vi "FDR.vi"(0 "System no.":i32=1 min=1 step=1, 1 "Board":i32=1 min=1 max=5 step=1, 2 "Routinename":string, 3 "Scan axis settings":T7={"Scan axis"="", "Range scan axis"=0.1, "Set Mid. pos?"=FALSE, "Mid. pos. scan axis"=0.1} {"Mid. pos. scan axis" format="%.4f"; "Range scan axis" format="%.4f"}, 4 "Step axis settings":T6={"Step axis"="", "Range step axis"=0.1, "Set Mid. pos?"=FALSE, "Mid. pos. step axis"=0.1} {"Mid. pos. step axis" format="%.4f"; "Range step axis" format="%.4f"}, 5 "error in":errorcluster, 6 "Threshold level":dbl=1.0 format="%.3f", 7 "Frequency settings":cluster{"Set frequency?":bool, "Frequency":dbl}={"Set frequency?"=FALSE, "Frequency"=10.0} {"Frequency" format="%.3f"}, 8 "Velocity settings":cluster{"Set velocity?":bool, "Velocity":dbl}={"Set velocity?"=FALSE, "Velocity"=0.1} {"Velocity" format="%.4f"}, 9 "Stop position option settings":T5, 10 "Target type settings":T4, 11 "Min. relative input level (MIIL) settings":T2={"Set min. input level?"=FALSE, "MIIL"=10.0}, 12 "Centroid method settings":T3, 13 "Max. relative input level (MAIL) settings":T1={"Set max. input level?"=FALSE, "MAIL"=80.0}) -> (19 "error out":errorcluster)   [LabVIEW 2026]
doc: "Defines a fast alignment area scan routine. Use FRS to start the routine and FRR? to read out the results of the routine. \n\nC-887, E-712, E-727.AS:"
panel:
  # "Defines a fast alignment raster scan routine. Use FRS to start the routine\nand FRR? to read out the results of the routine."
  # "If Yes:"
  # "If Yes:"
  # "If Yes:"
  # "If Yes:"
  # "If Yes:"
  # "If Yes:"
  # "If Yes:"
  # "If Yes:"
  # "If Yes:"
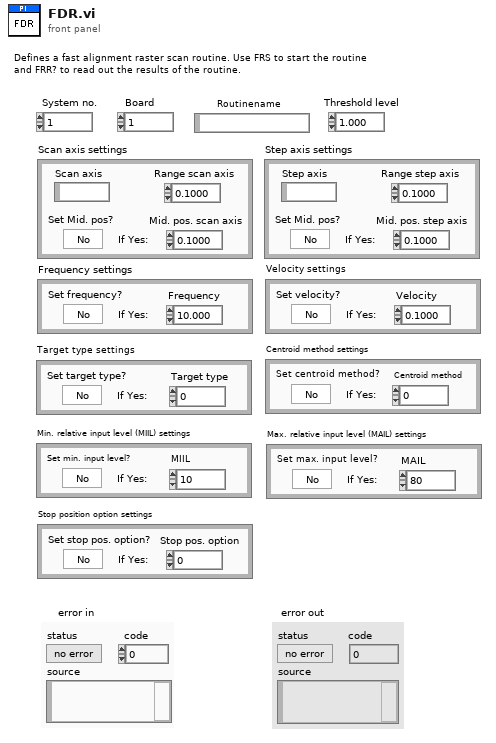
[diagram p1: front panel]
types:
  T1 = cluster{"Set max. input level?":bool, "MAIL":dbl}
  T2 = cluster{"Set min. input level?":bool, "MIIL":dbl}
  T3 = cluster{"Set centroid method?":bool, "Centroid method":i32}
  T4 = cluster{"Set target type?":bool, "Target type":i32}
  T5 = cluster{"Set stop pos. option?":bool, "Stop pos. option":i32}
  T6 = cluster{"Step axis":string, "Range step axis":dbl, "Set Mid. pos?":bool, "Mid. pos. step axis":dbl}
  T7 = cluster{"Scan axis":string, "Range scan axis":dbl, "Set Mid. pos?":bool, "Mid. pos. scan axis":dbl}
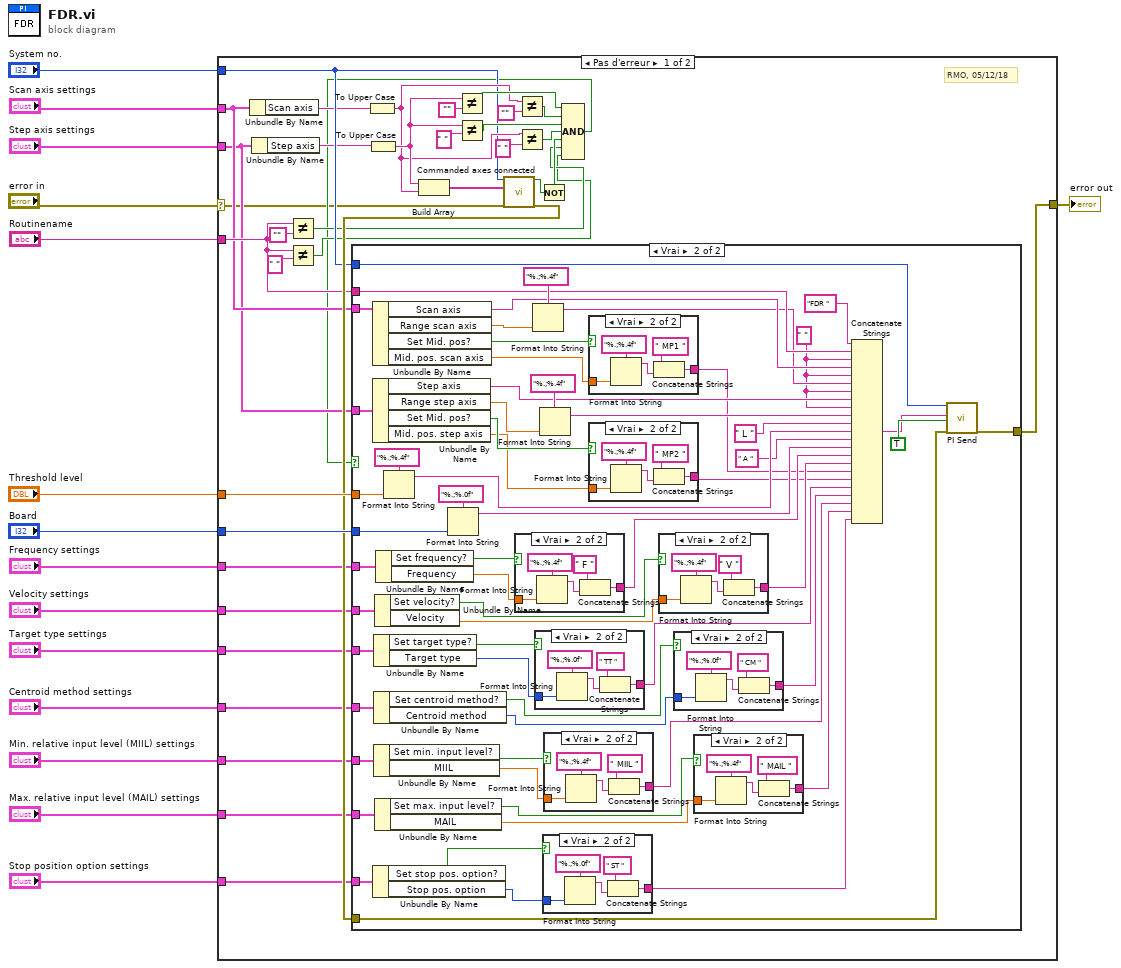
[diagram p0: block diagram]
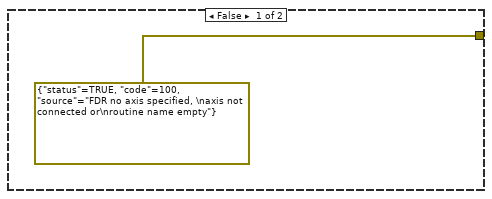
[diagram p2: hidden frame]
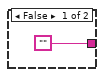
[diagram p3: hidden frame]
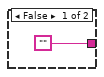
[diagram p4: hidden frame]
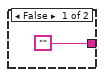
[diagram p5: hidden frame]
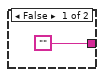
[diagram p6: hidden frame]
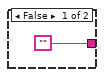
[diagram p7: hidden frame]
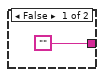
[diagram p8: hidden frame]
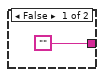
[diagram p9: hidden frame]
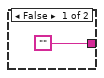
[diagram p10: hidden frame]
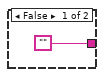
[diagram p11: hidden frame]
diagram:
  n1 = case shown="Pas d'erreur" "error in" {
    selector: "error in" -> [w16 w167]
    tunnel: "System no." -> [w34 _]
    tunnel: [w44 w167] -> w14
    tunnel: "Step axis settings" -> [w25 _]
    tunnel: "Board" -> [w47 _]
    tunnel: "Velocity settings" -> [w23 _]
    tunnel: "Stop position option settings" -> [w22 _]
    tunnel: "Threshold level" -> [w46 _]
    tunnel: "Scan axis settings" -> [w26 _]
    tunnel: "Routinename" -> [w27 _]
    tunnel: "Frequency settings" -> [w24 _]
    tunnel: "Target type settings" -> [w21 _]
    tunnel: "Centroid method settings" -> [w20 _]
    tunnel: "Min. relative input level (MIIL) settings" -> [w19 _]
    tunnel: "Max. relative input level (MAIL) settings" -> [w18 _]
    frame No Error {
      # "RMO, 05/12/18"
      n2 = Unbundle By Name(w26) -> ("Scan axis"=w33:string)
      n3 = Unbundle By Name(w25) -> ("Step axis"=w32:string)
      n4 = Not Equal?(x=w27, y="") -> (x != y?=w29:bool)
      n5 = Not Equal?(x=w27, y=" ") -> (x != y?=w28:bool)
      n6 = To Upper Case(1:w33) -> (0:w35:string)
      n7 = To Upper Case(1:w32) -> (0:w36:string)
      n8 = Build Array(w36, w35) -> (w48:string[])
      n9 = Not Equal?(x=w36, y="") -> (x != y?=w49:bool)
      n10 = Not Equal?(x=w36, y=" ") -> (x != y?=w39:bool)
      n11 = call "Commanded axes connected.vi"("System no."=w34, "Commanded axes"=w48, "error in"=w16) -> ("Controller error"=w43:bool, "error out"=w45:errorcluster)  [unwired: 15 out]
      n12 = Not Equal?(x=w35, y="") -> (x != y?=w38:bool)
      n13 = Not Equal?(x=w35, y=" ") -> (x != y?=w37:bool)
      n14 = Not(x=w43) -> (.not. x?=w42:bool)
      n15 = Compound Arithmetic op=AND(w49, w38, w39, w37, w42, w29, w28) -> (w17:bool)
      n16 = case shown="Vrai" w17 {
        tunnel: w47 -> [_ w103]
        tunnel: w46 -> [_ w92]
        tunnel: w45 -> [_ w112]
        tunnel: w34 -> [_ w105]
        tunnel: [errorcluster {"status"=TRUE, "code"=100, "source"="FDR no axis specified, \naxis not connected or\nroutine name empty"} ("error out") w53] -> w44
        tunnel: w27 -> [_ w101]
        tunnel: w26 -> [_ w100]
        tunnel: w25 -> [_ w96]
        tunnel: w24 -> [_ w87]
        tunnel: w23 -> [_ w71]
        tunnel: w22 -> [_ w74]
        tunnel: w21 -> [_ w70]
        tunnel: w20 -> [_ w69]
        tunnel: w19 -> [_ w68]
        tunnel: w18 -> [_ w67]
        frame False {
        }
        frame True {
          w93 = " "
          n17 = Unbundle By Name(w100) -> ("Scan axis"=w99:string, "Range scan axis"=w98:dbl, "Set Mid. pos?"=w82:bool, "Mid. pos. scan axis"=w78:dbl)
          n18 = Unbundle By Name(w96) -> ("Step axis"=w95:string, "Range step axis"=w94:dbl, "Set Mid. pos?"=w81:bool, "Mid. pos. step axis"=w77:dbl)
          n19 = Unbundle By Name(w74) -> ("Set stop pos. option?"=w73:bool, "Stop pos. option"=w72:i32)
          n20 = Unbundle By Name(w70) -> ("Set target type?"=w66:bool, "Target type"=w65:i32)
          n21 = Unbundle By Name(w69) -> ("Set centroid method?"=w54:bool, "Centroid method"=w63:i32)
          n22 = Unbundle By Name(w68) -> ("Set min. input level?"=w61:bool, "MIIL"=w60:dbl)
          n23 = Unbundle By Name(w71) -> ("Set velocity?"=w84:bool, "Velocity"=w79:dbl)
          n24 = Unbundle By Name(w67) -> ("Set max. input level?"=w58:bool, "MAIL"=w57:dbl)
          n25 = Unbundle By Name(w87) -> ("Set frequency?"=w86:bool, "Frequency"=w80:dbl)
          n26 = Format Into String(format string="%.;%.4f" ("Format String"), w92) -> (resulting string=w90:string)  [unwired: 2 in, 1 out]
          n27 = Format Into String(format string="%.;%.0f" ("Format String"), w103) -> (resulting string=w88:string)  [unwired: 2 in, 1 out]
          n28 = case shown="Vrai" w86 {
            tunnel: ["" w163] -> w85
            tunnel: w80 -> [_ w162]
            frame False {
            }
            frame True {
              n29 = Format Into String(format string="%.;%.4f" ("Format String"), w162) -> (resulting string=w164:string)  [unwired: 2 in, 1 out]
              n30 = Concatenate Strings(" F ", w164) -> (w163:string)
            }
          }
          n31 = Format Into String(format string="%.;%.4f" ("Format String"), w98) -> (resulting string=w97:string)  [unwired: 2 in, 1 out]
          n32 = case shown="Vrai" w66 {
            tunnel: ["" w133] -> w64
            tunnel: w65 -> [_ w132]
            frame False {
            }
            frame True {
              n33 = Format Into String(format string="%.;%.0f" ("Format String"), w132) -> (resulting string=w134:string)  [unwired: 2 in, 1 out]
              n34 = Concatenate Strings(" TT ", w134) -> (w133:string)
            }
          }
          n35 = Format Into String(format string="%.;%.4f" ("Format String"), w94) -> (resulting string=w107:string)  [unwired: 2 in, 1 out]
          n36 = case shown="Vrai" w73 {
            tunnel: ["" w139] -> w55
            tunnel: w72 -> [_ w138]
            frame False {
            }
            frame True {
              n37 = Format Into String(format string="%.;%.0f" ("Format String"), w138) -> (resulting string=w140:string)  [unwired: 2 in, 1 out]
              n38 = Concatenate Strings(" ST ", w140) -> (w139:string)
            }
          }
          n39 = case shown="Vrai" w61 {
            tunnel: ["" w121] -> w59
            tunnel: w60 -> [_ w120]
            frame False {
            }
            frame True {
              n40 = Format Into String(format string="%.;%.4f" ("Format String"), w120) -> (resulting string=w122:string)  [unwired: 2 in, 1 out]
              n41 = Concatenate Strings(" MIIL ", w122) -> (w121:string)
            }
          }
          n42 = case shown="Vrai" w82 {
            tunnel: ["" w151] -> w76
            tunnel: w78 -> [_ w150]
            frame False {
            }
            frame True {
              n43 = Format Into String(format string="%.;%.4f" ("Format String"), w150) -> (resulting string=w152:string)  [unwired: 2 in, 1 out]
              n44 = Concatenate Strings(" MP1 ", w152) -> (w151:string)
            }
          }
          n45 = case shown="Vrai" w81 {
            tunnel: ["" w145] -> w75
            tunnel: w77 -> [_ w144]
            frame False {
            }
            frame True {
              n46 = Format Into String(format string="%.;%.4f" ("Format String"), w144) -> (resulting string=w146:string)  [unwired: 2 in, 1 out]
              n47 = Concatenate Strings(" MP2 ", w146) -> (w145:string)
            }
          }
          n48 = case shown="Vrai" w84 {
            tunnel: ["" w157] -> w83
            tunnel: w79 -> [_ w156]
            frame False {
            }
            frame True {
              n49 = Format Into String(format string="%.;%.4f" ("Format String"), w156) -> (resulting string=w158:string)  [unwired: 2 in, 1 out]
              n50 = Concatenate Strings(" V ", w158) -> (w157:string)
            }
          }
          n51 = case shown="Vrai" w54 {
            tunnel: ["" w127] -> w62
            tunnel: w63 -> [_ w126]
            frame False {
            }
            frame True {
              n52 = Format Into String(format string="%.;%.0f" ("Format String"), w126) -> (resulting string=w128:string)  [unwired: 2 in, 1 out]
              n53 = Concatenate Strings(" CM ", w128) -> (w127:string)
            }
          }
          n54 = case shown="Vrai" w58 {
            tunnel: ["" w115] -> w56
            tunnel: w57 -> [_ w114]
            frame False {
            }
            frame True {
              n55 = Format Into String(format string="%.;%.4f" ("Format String"), w114) -> (resulting string=w116:string)  [unwired: 2 in, 1 out]
              n56 = Concatenate Strings(" MAIL ", w116) -> (w115:string)
            }
          }
          n57 = Concatenate Strings("FDR ", w101, w93, w99, w93, w97, w93, w95, w93, w107, " L ", w90, " A ", w88, w85, w83, w76, w75, w64, w62, w59, w56, w55) -> (w102:string)
          n58 = call "PI Send.vi"("System no."=w105, "String to send"=w102, "Attach termination char.?"=TRUE ("Attach Linefeed?"), "error in"=w112) -> ("error out"=w53:errorcluster)  [unwired: 2 in, 13 out]
        }
      }
    }
    frame Error {
    }
  }
  "error out" <- w14
